vi "Read RP Level Configuration.vi"(8 "error in (no error)":errorcluster, 11 "RP Delayed in":refnum<class "RP Level.lvclass">) -> (0 "error out":errorcluster, 2 "RP Delayed Configuration":T1={"Pre-trigger duration"=0.01, "Post-trigger duration"=0.1, "Rate"=1000000.0, "Ranges"=[10.0], "Re-name channels"=[], "Active channels"="0:1", "External clock"=FALSE, "Output delay"=0.1, "Raising edge "=FALSE, "Trigger level"=0.001} {"Trigger level" format="%#_6pV"; "Output delay" format="%#_6ps"; "Rate" format="%#_8pHz"; "Post-trigger duration" format="%#_6ps"; "Pre-trigger duration" format="%#_6ps"; "Ranges" format="%#_6pV"}, 3 "RP Delayed out":refnum<class "RP Level.lvclass">)   [LabVIEW 2018, in "RP Level.lvclass"]
uses:
  RP Level.lvclass
  C:/github/LabActor/Template Module/Template Module.lvclass
  NHMFL_Core/Libraries/Red Pitaya/RP Level Configuration.ctl
  Template Module/Template Module.lvclass/Template Module.ctl
  Template Module/Read Configuration.vi
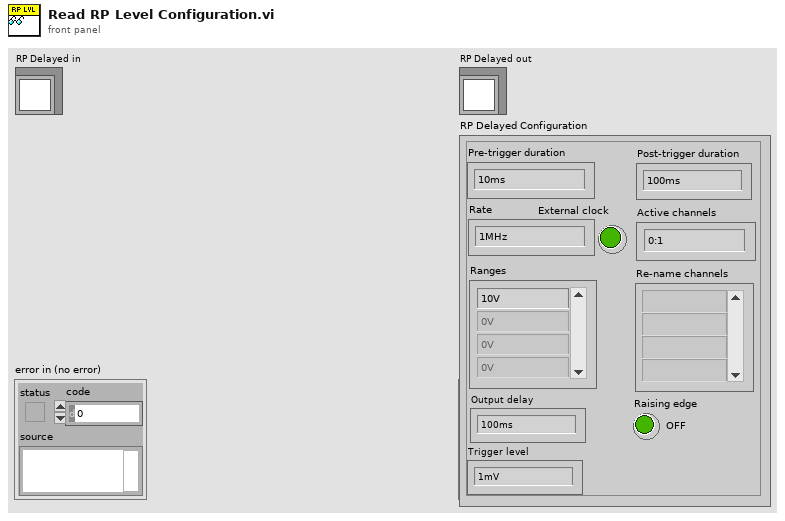
[diagram p1: front panel]
types:
  T1 = typedef "RP Level Configuration.ctl" = cluster{"Pre-trigger duration":dbl, "Post-trigger duration":dbl, "Rate":dbl, "Ranges":dbl[], "Re-name channels":string[], "Active channels":string, "External clock":bool, "Output delay":dbl, "Raising edge ":bool, "Trigger level":dbl}
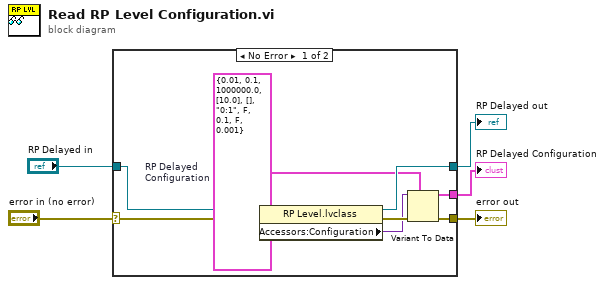
[diagram p0: block diagram]
diagram:
  n1 = case shown="No Error" "error in (no error)" {
    selector: "error in (no error)" -> [w13 w14]
    tunnel: [w9 w14] -> w4
    tunnel: [w11 w15] -> w2
    tunnel: "RP Delayed in" -> [w12 w15]
    tunnel: [w6 _] -> w1
    frame No Error {
      w7 = T1 {"Pre-trigger duration"=0.01, "Post-trigger duration"=0.1, "Rate"=1000000.0, "Ranges"=[10.0], "Re-name channels"=[], "Active channels"="0:1", "External clock"=FALSE, "Output delay"=0.1, "Raising edge "=FALSE, "Trigger level"=0.001}  # RP Delayed Configuration
      n2 = property class="RP Level.lvclass"(reference=w12, error in=w13) -> (reference out=w11:refnum<class "RP Level.lvclass">, error out=w10:errorcluster, "Accessors:Configuration"=w8:variant)
      n3 = Variant To Data(error in=w10, type=w7, Variant=w8) -> (data=w6:T1, error out=w9:errorcluster)
    }
    frame Error {
    }
  }
  "error out" <- w4
  "RP Delayed out" <- w2
  "RP Delayed Configuration" <- w1
